vi "格式化写入文本文件.vi"() -> ()   [LabVIEW 2010]
panel:
  in  "记录数据":bool
  in  "停止":bool
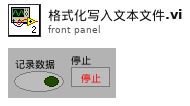
[diagram p1: front panel]
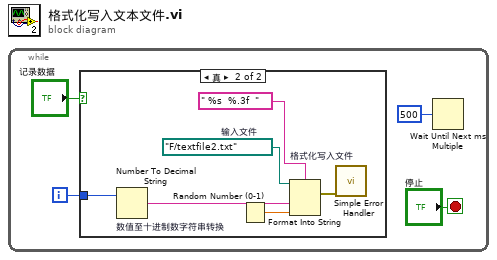
[diagram p0: block diagram]
diagram:
  n1 = while {
    i -> [w2]
    stop <- "停止" stop-if-true
    n2 = case shown="真" "记录数据" {
      tunnel: w2 -> [_ w7]
      frame False {
      }
      frame True {
        w10 = path "F:/textfile2.txt"  # 输入文件
        n3 = Number To Decimal String "数值至十进制数字符串转换"(number=w7) -> (decimal integer string=w6:string)  [unwired: 1 in]
        n4 = Random Number (0-1)() -> (number: 0 to 1=w8:dbl)
        n5 = Format Into String "格式化写入文件"(format string=" %s  %.3f  " ("格式字符串"), initial string=w10, w6, w8) -> (error out=w5:errorcluster)  [unwired: 1 in, 1 out]
        n6 = call <vilib>:"Simple Error Handler.vi"("error in (no error)"=w5) -> ()  [unwired: 4 in, 5 out]
      }
    }
    n7 = Wait Until Next ms Multiple(millisecond multiple=u32 500 ("毫秒倍数")) -> ()  [unwired: 1 out]
  }
